vi "ChannelType_1D-Array-3DPoint-DBL.vi"(9 "error in":errorcluster, 11 "Array in":T1[](array[typedef])) -> (1 "error out":errorcluster, 2 "ChannelType":dbl, 3 "Array out":T1[](array[typedef]))   [LabVIEW 2020, in "OpenLvVision_OpenCv.lvlib"]
uses:
  OpenLvVision_OpenCv.lvlib
  TypeDef/Point/3D_PointDBL.ctl
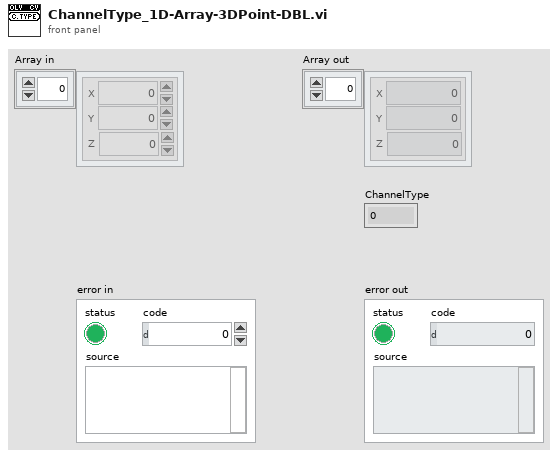
[diagram p1: front panel]
types:
  T1 = typedef "OpenLvVision_OpenCv.lvlib/3D_PointDBL.ctl" = cluster{"X":dbl, "Y":dbl, "Z":dbl}
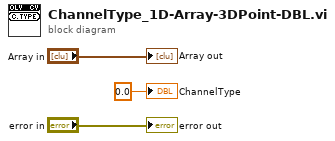
[diagram p0: block diagram]
diagram:
  "error out" <- "error in"
  "Array out" <- "Array in"
  "ChannelType" <- 0.0
